vi "FGV Daten Regler.vi"(6 "Aktionen":T2, 10 "PID - OUT%":T1, 11 "Heizung EIN":bool) -> (2 "PID - OUT%":T1, 3 "Heizung EIN":bool)   [LabVIEW 2020, in "Regler.lvlib"]
uses:
  Regler.lvlib
  FGV Daten Regler Aktionen.ctl
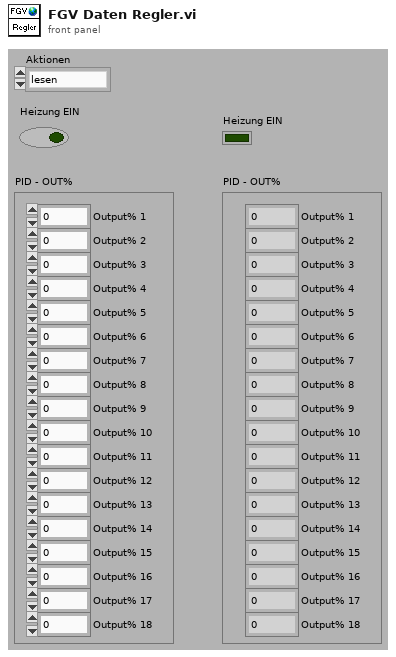
[diagram p1: front panel]
types:
  T1 = cluster{"Output% 1":i16, "Output% 2":i16, "Output% 3":i16, "Output% 4":i16, "Output% 5":i16, "Output% 6":i16, "Output% 7":i16, "Output% 8":i16, "Output% 9":i16, "Output% 10":i16, "Output% 11":i16, "Output% 12":i16, "Output% 13":i16, "Output% 14":i16, "Output% 15":i16, "Output% 16":i16, "Output% 17":i16, "Output% 18":i16}
  T2 = typedef "Regler.lvlib/FGV Daten Regler Aktionen.ctl" = enum16{"lesen", "Out%", "Heizung EIN"}
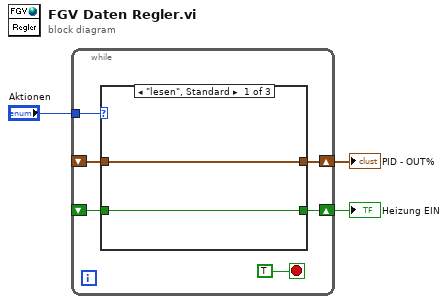
[diagram p0: block diagram]
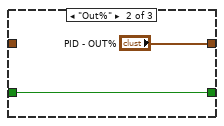
[diagram p2: hidden frame]
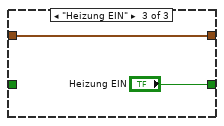
[diagram p3: hidden frame]
diagram:
  n1 = while {
    tunnel: "Aktionen" -> [w8]
    shift-right: [w6] -> w2
    shift-left: _ -> [w7]
    shift-right: [w4] -> w1
    shift-left: _ -> [w5]
    stop <- TRUE stop-if-true
    n2 = case shown="\"lesen\", Standard" w8 {
      tunnel: w7 -> [w11 _ w14]
      tunnel: [w11 "PID - OUT%" w14] -> w6
      tunnel: w5 -> [w10 w12 _]
      tunnel: [w10 w12 "Heizung EIN"] -> w4
      frame "lesen", Default {
      }
      frame "Out%" {
      }
      frame "Heizung EIN" {
      }
    }
  }
  "PID - OUT%" <- w2
  "Heizung EIN" <- w1
